vi "pan track.vi"(7 "Knob":dbl, 11 "Track In":T1) -> (3 "Track Out":T1)   [LabVIEW 2014]
uses:
  Controls/Audio In.ctl
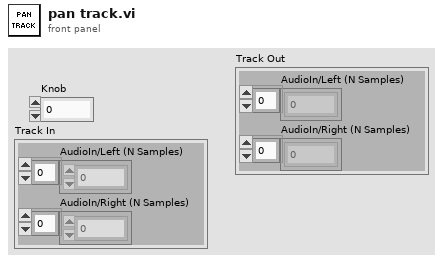
[diagram p1: front panel]
types:
  T1 = typedef "Audio In.ctl" = cluster{"AudioIn/Left (N Samples)":dbl[], "AudioIn/Right (N Samples)":dbl[]}
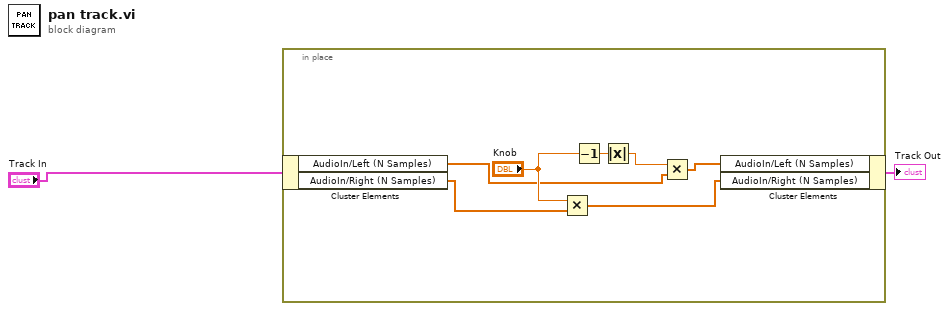
[diagram p0: block diagram]
diagram:
  n1 = in-place {
    n2 = in-place-cluster #1("Track In") -> ("AudioIn/Left (N Samples)"=w6:dbl[], "AudioIn/Right (N Samples)"=w4:dbl[])
    n3 = Multiply(x="Knob", y=w4) -> (x*y=w3:dbl[])
    n4 = Decrement(x="Knob") -> (x-1=w8:dbl)
    n5 = Absolute Value(x=w8) -> (abs(x)=w9:dbl)
    n6 = Multiply(x=w9, y=w6) -> (x*y=w5:dbl[])
    n7 = in-place-cluster #1("AudioIn/Left (N Samples)"=w5, "AudioIn/Right (N Samples)"=w3) -> (→"Track Out":T1)
  }
